vi "FGEN Function Generator.vi"() -> ()   [LabVIEW 2021]
doc: "This example shows the Standard Function output mode. \n\nIt also shows some of the parameters which can be changed on the fly."
uses:
  <instrlib>/niFgen/niFgen.llb/niFgen Output Mode.ctl
panel:
  in  "Standard Waveform":u16(slide) scale=0.0..6.0
  in  "Start Phase":dbl
  in  "Stop":bool
  in  "FGEN Resource Name":refnum<k15>="FGEN0"
  in  "DC Offset (V)":dbl(knob) min=-6.0 max=6.0 scale=-6.0..6.0 scale format="%_1p"
  in  "Frequency (Hz)":dbl(knob)=1000000.0 min=9000.0 max=100000000.0 scale=0.0..100000000.0 scale format="%_1p"
  in  "Amplitude (Vp-p)":dbl(knob)=1.0 min=0.0 max=12.0 scale=0.0..12.0 scale format="%.1f"
  # "Overview: Demonstrates the Standard Function output mode for NI Function Generators. It also shows some of the parameters which can be changed on the fly.\nSoftware Requirements: NI-FGEN\nHardware Requirements: PXI-5401, PCI-5401, PXI-5402, PCI-5402, PXI-5406, PCI-5406, PXI-5411, PCI-5411, AT-5411, PXI-5412, PCI-5412, PXIe-5413, PXI-5421, PCI-5421, PXI-5422, PXIe-5423, PXI-5431, PCI-5431, PXIe-5433, PXI-5441, NI PXIe-5442, NI PXIe-5450, or NI PXIe-5451 \nInstructions:\n1. Select the FGEN Resource Name as configured in the Measurement & Automation Explorer.\n2. Select the Standard Waveform that will be generated.\n3. Specify the Amplitude (Vp-p) that will be used.\n4. Specify the Frequency (Hz) that will be used\n5. Specify the DC Offset (V) that will be used\n6. Run the VI.\n7. You can change the Amplitude (Vp-p), Frequency (Hz), or DC Offset (V) values on-the-fly.\n8. Click Stop to stop the VI."
  # "<-- must manutally enter, FGen device will not be found\nin drop down"
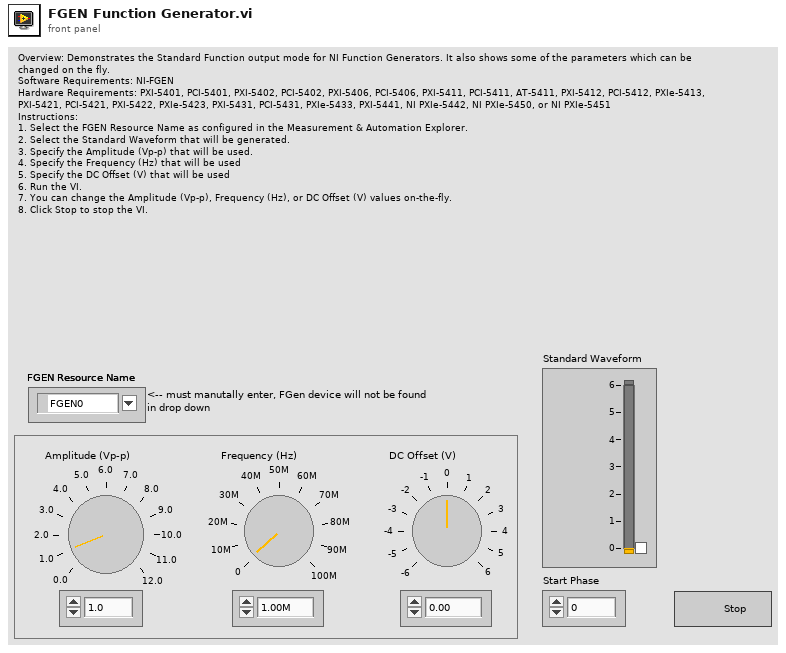
[diagram p1: front panel]
types:
  T1 = typedef "niFgen Output Mode.ctl" = u32
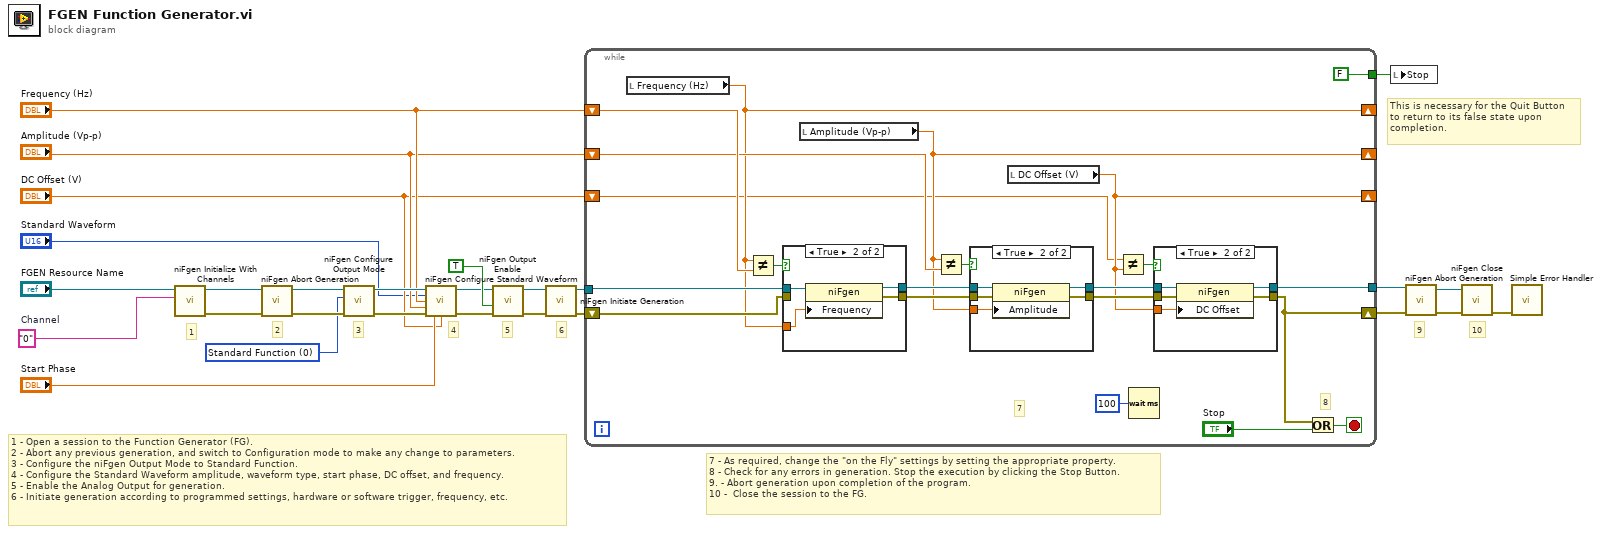
[diagram p0: block diagram]
diagram:
  w17 = T1 0 items=["Standard Function", "Frequency List", "Arbitrary Waveform", "Arbitrary Sequence", "Script"] ("output mode")
  w1 = "0"  # Channel
  # "This is necessary for the Quit Button\nto return to its false state upon\ncompletion."
  # "10"
  # "9"
  # "7 - As required, change the \"on the Fly\" settings by setting the appropriate property. \n8 - Check for any errors in generation. Stop the execution by clicking the Stop Button.\n9. - Abort generation upon completion of the program.\n10 -  Close the session to the FG."
  # "6"
  # "5"
  # "4"
  # "3"
  # "2"
  # "1"
  # "1 - Open a session to the Function Generator (FG).\n2 - Abort any previous generation, and switch to Configuration mode to make any change to parameters.\n3 - Configure the niFgen Output Mode to Standard Function.\n4 - Configure the Standard Waveform amplitude, waveform type, start phase, DC offset, and frequency.\n5 - Enable the Analog Output for generation.\n6 - Initiate generation according to programmed settings, hardware or software trigger, frequency, etc."
  n1 = call <instrlib>:"niFgen Initialize With Channels.vi"("Channel Name"=w1, "Resource Name"="FGEN Resource Name") -> ("error out"=w4:errorcluster, "Instrument Handle Out"=w3:refnum<k15>)  [unwired: 8 in]
  n2 = call <instrlib>:"niFgen Abort Generation.vi"("error in (no error)"=w4, "Instrument Handle"=w3) -> ("error out"=w20:errorcluster, "Instrument Handle Out"=w19:refnum<k15>)  [unwired: 8 in]
  n3 = call <instrlib>:"niFgen Configure Output Mode.vi"("error in (no error)"=w20, "Output Mode (default: 0=Standard Function)"=w17, "Instrument Handle"=w19) -> ("error out"=w24:errorcluster, "Instrument Handle Out"=w22:refnum<k15>)  [unwired: 6 in]
  n4 = call <instrlib>:"niFgen Configure Standard Waveform.vi"("Instrument Handle"=w22, "Waveform"="Standard Waveform", "Frequency"="Frequency (Hz)", "Amplitude"="Amplitude (Vp-p)", "error in (no error)"=w24, "Start Phase"="Start Phase", "DC Offset"="DC Offset (V)") -> ("Instrument Handle Out"=w15:refnum<k15>, "error out"=w16:errorcluster)  [unwired: 7 in]
  n5 = call <instrlib>:"niFgen Output Enable.vi"("error in (no error)"=w16, "Output Enable (default: True)"=TRUE ("output enable"), "Instrument Handle"=w15) -> ("error out"=w23:errorcluster, "Instrument Handle Out"=w21:refnum<k15>)  [unwired: 7 in]
  n6 = call <instrlib>:"niFgen Initiate Generation.vi"("error in (no error)"=w23, "Instrument Handle"=w21) -> ("error out"=w9:errorcluster, "Instrument Handle Out"=w13:refnum<k15>)  [unwired: 8 in]
  n7 = while {
    tunnel: w13 -> [w43]
    tunnel: [w44] -> w12
    shift-right: [w32] -> _
    shift-left: "Frequency (Hz)" -> [w41]
    shift-right: [w31] -> _
    shift-left: "Amplitude (Vp-p)" -> [w40]
    shift-right: [w30] -> _
    shift-left: "DC Offset (V)" -> [w29]
    shift-right: [w33] -> w8
    shift-left: w9 -> [w42]
    tunnel: [FALSE] -> w5
    stop <- w34 stop-if-true
    # "8"
    # "7"
    n8 = local read "Frequency (Hz)"() -> (w32:dbl)
    n9 = Not Equal?(x=w32, y=w41) -> (x != y?=w39:bool)
    n10 = case shown="True" w39 {
      tunnel: [w64 w68] -> w45
      tunnel: [w63 w67] -> w46
      tunnel: w43 -> [w64 w66]
      tunnel: w42 -> [w63 _]
      tunnel: w32 -> [_ w65]
      frame False {
      }
      frame True {
        n11 = property class="niFgen"(reference=w66, "Frequency"=w65) -> (reference out=w68:refnum<k15>, error out=w67:errorcluster)  [unwired: 1 in]
      }
    }
    n12 = local read "Amplitude (Vp-p)"() -> (w31:dbl)
    n13 = Not Equal?(x=w31, y=w40) -> (x != y?=w38:bool)
    n14 = case shown="True" w38 {
      tunnel: w45 -> [w57 w62]
      tunnel: w46 -> [w56 w61]
      tunnel: [w56 w60] -> w47
      tunnel: [w57 w59] -> w48
      tunnel: w31 -> [_ w58]
      frame False {
      }
      frame True {
        n15 = property class="niFgen"(reference=w62, error in=w61, "Amplitude"=w58) -> (reference out=w59:refnum<k15>, error out=w60:errorcluster)
      }
    }
    n16 = local read "DC Offset (V)"() -> (w30:dbl)
    n17 = Not Equal?(x=w29, y=w30) -> (x != y?=w37:bool)
    n18 = Wait (ms)(milliseconds to wait=u32 100) -> ()  [unwired: 1 out]
    n19 = case shown="True" w37 {
      tunnel: w47 -> [w49 w55]
      tunnel: w48 -> [w50 w54]
      tunnel: [w50 w53] -> w44
      tunnel: [w49 w52] -> w33
      tunnel: w30 -> [_ w51]
      frame False {
      }
      frame True {
        n20 = property class="niFgen"(reference=w54, error in=w55, "DC Offset"=w51) -> (reference out=w53:refnum<k15>, error out=w52:errorcluster)
      }
    }
    n21 = Or(x=w33, y="Stop") -> (x .or. y?=w34:bool)
  }
  n22 = local write "Stop"(w5) -> ()
  n23 = call <instrlib>:"niFgen Abort Generation.vi"("error in (no error)"=w8, "Instrument Handle"=w12) -> ("error out"=w26:errorcluster, "Instrument Handle Out"=w27:refnum<k15>)  [unwired: 8 in]
  n24 = call <instrlib>:"niFgen Close.vi"("error in (no error)"=w26, "Instrument Handle"=w27) -> ("error out"=w25:errorcluster)  [unwired: 9 in]
  n25 = call <vilib>:"Simple Error Handler.vi"("error in (no error)"=w25) -> ()  [unwired: 4 in, 5 out]
